vi "Multiple_ROIs.vi"() -> ()   [LabVIEW 2018]
panel:
  out "ROI":T1
  in  "File Path":path
  in  "Stop":bool
  out "Image Display":T2(plugin-control)
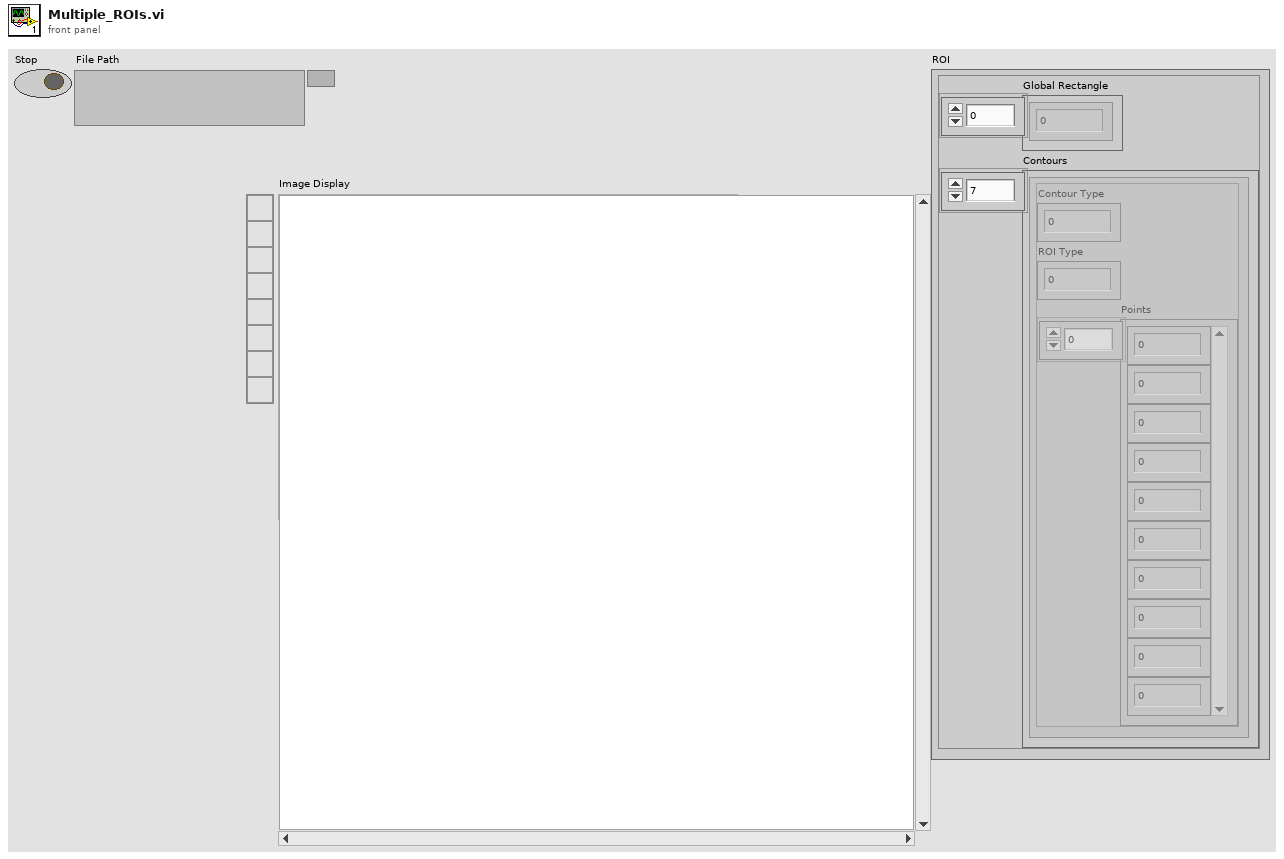
[diagram p1: front panel]
types:
  T1 = cluster{"Global Rectangle":i32[], "Contours":cluster{"Contour Type":u32, "ROI Type":u32, "Points":i32[]}[]}
  T2 = typedef "IMAQ Image.ctl" = refnum<image>
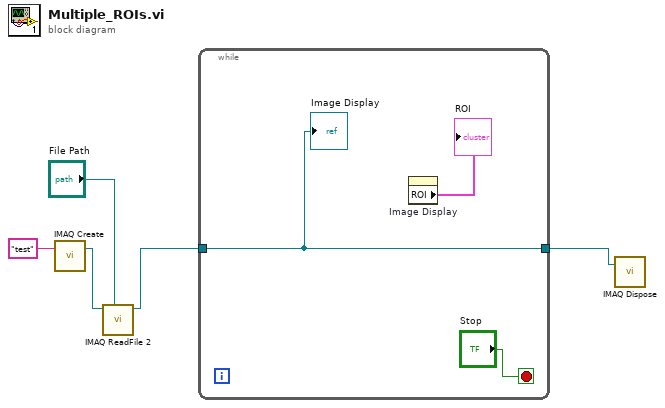
[diagram p0: block diagram]
diagram:
  n1 = call "IMAQ Create"("Image Name"="test") -> ("New Image"=w3:T2)  [unwired: 4 in, 1 out]
  n2 = call "IMAQ ReadFile 2"("File Path"="File Path", "Image"=w3) -> ("Image Out"=w2:T2)  [unwired: 5 in, 4 out]
  n3 = while {
    tunnel: w2 -> [w7]
    tunnel: [w7] -> w4
    stop <- "Stop" stop-if-true
    n4 = property on="Image Display" class="ImageControl"() -> ("ROI"=→"ROI":T1)  [unwired: 2 in, 2 out]
    "Image Display" <- w7
  }
  n5 = call "IMAQ Dispose"("Image"=w4) -> ()  [unwired: 5 in, 1 out]
